vi "Get Alias_Do.vi"(8 "error in (no error)":errorcluster, 11 "Project Action in":refnum<class "Project Action.lvclass">) -> (0 "error out":errorcluster, 2 "Alias":string, 3 "Project Action out":refnum<class "Project Action.lvclass">)   [LabVIEW 2020, in "ProjectBuilder.lvlib" / "Project Action.lvclass"]
uses:
  Project Action.lvclass
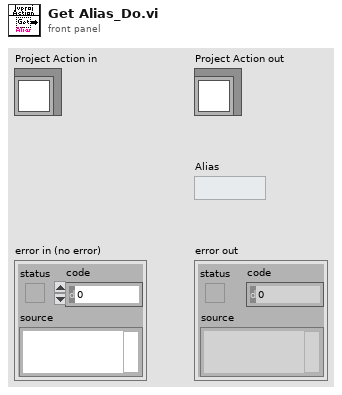
[diagram p1: front panel]
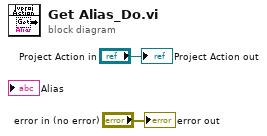
[diagram p0: block diagram]
diagram:
  "error out" <- "error in (no error)"
  "Project Action out" <- "Project Action in"
